vi "service_error_parse.vi"(0 "Reply":string="\u0000\u0000\u0000\u0000\u0000") -> (1 "OK?":bool, 2 "Error Code":i32)   [LabVIEW 2013]
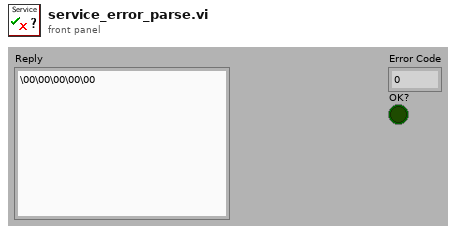
[diagram p1: front panel]
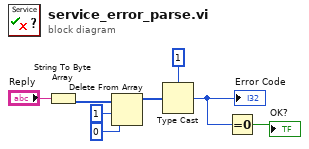
[diagram p0: block diagram]
diagram:
  n1 = String To Byte Array(string="Reply") -> (unsigned byte array=w7:u8[])
  n2 = Delete From Array(array=w7, length=1, index=0) -> (array with subset deleted=w4:u8[])  [unwired: 1 out]
  n3 = Type Cast(type=1 ("length"), x=w4) -> (*(type *) &x=w2:i32)
  "Error Code" <- w2
  n4 = Equal To 0?(x=w2) -> (x = 0?=→"OK?":bool)
